vi "Gyro Reset.vi"(11 "I2CDevRef":T1 {"Device Address" format="%.0x"}) -> (3 "I2CDevRef Out":T1 {"Device Address" format="%.0x"})   [LabVIEW 2013]
uses:
  <vilib>/Rock Robotics/WPI/I2C/WPI_I2CDevRef.ctl
  <vilib>/Rock Robotics/SystemInterfaces/Typedef/FPGA_TypedefDigitalModule.ctl
  Gyro Globals.vi
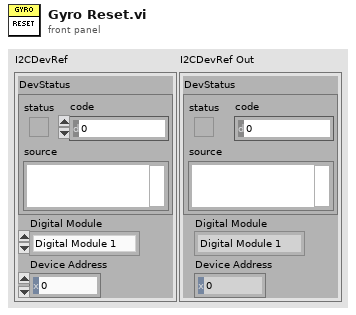
[diagram p1: front panel]
types:
  T1 = typedef "WPI_I2CDevRef.ctl" = cluster{"DevStatus":errorcluster, "Digital Module":T2, "Device Address":u8}
  T2 = typedef "FPGA_TypedefDigitalModule.ctl" = enum16{"Digital Module 1", "Digital Module 2"}
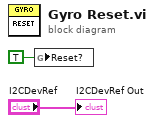
[diagram p0: block diagram]
diagram:
  n1 = global write "Gyro Globals.vi" "Reset?"(TRUE ("Reset?")) -> ()
  "I2CDevRef Out" <- "I2CDevRef"
